vi "DBAL-constructor.vi"(8 "error in (no error)":errorcluster, 11 "DBAL in":refnum<class "DBAL.lvclass">) -> (0 "error out":errorcluster, 3 "DBAL out":refnum<class "DBAL.lvclass">)   [LabVIEW 2020, in "Sgraph_lib_V1.lvlib" / "DBAL.lvclass"]
doc: "Constructor of the DBAL service.\n\nThe DBAL service must take care that file save actions do not cost valuable time that is needed for maximum graph responsiveness.\nTherefore DB write actions must be buffered, while DB read actions can be performed immediate.\nIf possible: simultaneously."
uses:
  DBAL.lvclass
  DBAL.lvclass/DBAL.ctl
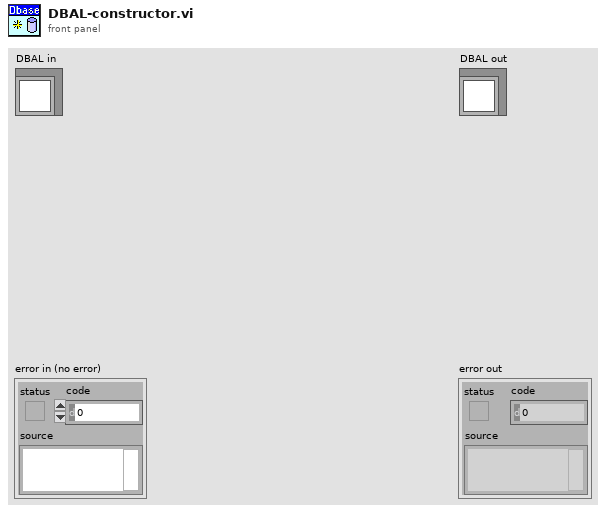
[diagram p1: front panel]
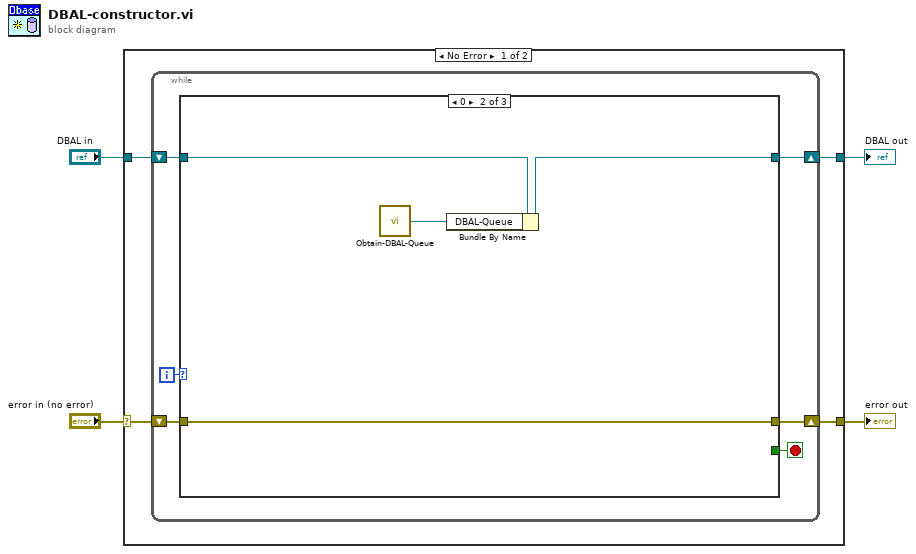
[diagram p0: block diagram]
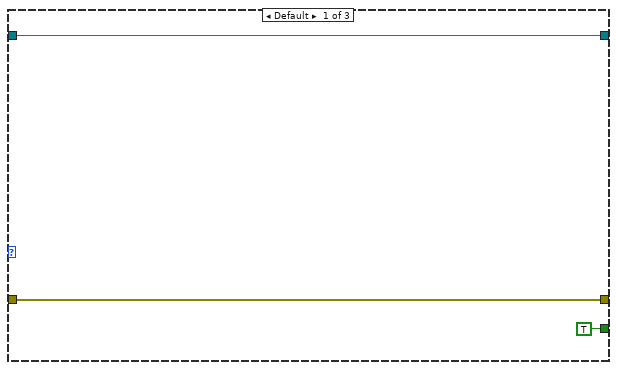
[diagram p2: hidden frame]
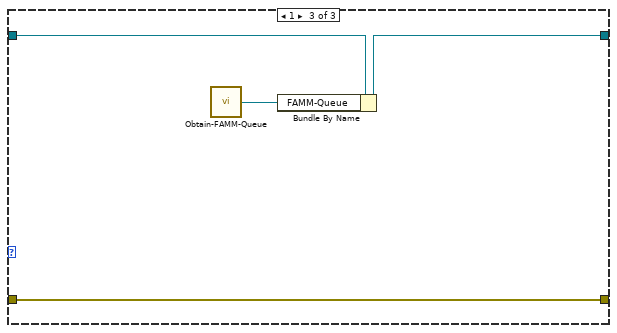
[diagram p3: hidden frame]
diagram:
  n1 = case shown="No Error" "error in (no error)" {
    selector: "error in (no error)" -> [w7 w26]
    tunnel: [w7 w26] -> w3
    tunnel: [w5 w25] -> w1
    tunnel: "DBAL in" -> [w6 w25]
    frame No Error {
      n2 = while {
        shift-right: [w11] -> _
        shift-left: w7 -> [w13]
        shift-right: [w8] -> w5
        shift-left: w6 -> [w9]
        i -> [w12]
        stop <- w10 stop-if-true
        n3 = case shown="0" w12 {
          tunnel: w13 -> [w16 w17 w21]
          tunnel: [w16 w17 w21] -> w11
          tunnel: [TRUE _ _] -> w10
          tunnel: w9 -> [w14 w19 w24]
          tunnel: [w14 w20 w22] -> w8
          frame Default {
          }
          frame 0 {
            n4 = call "Obtain-DBAL-Queue.vi"() -> ("DBAL-Queue"=w18:refnum<queue>)  [unwired: 7 in]
            n5 = Bundle By Name(cluster=w19, "DBAL-Queue"=w18) -> (w20:refnum<class "DBAL.lvclass">)
          }
          frame 1 {
            n6 = call "Obtain-FAMM-Queue.vi"() -> ("FAMM-Queue"=w23:refnum<queue>)  [unwired: 7 in]
            n7 = Bundle By Name(cluster=w24, "FAMM-Queue"=w23) -> (w22:refnum<class "DBAL.lvclass">)
          }
        }
      }
    }
    frame Error {
    }
  }
  "error out" <- w3
  "DBAL out" <- w1
